vi "classify error.vi"(8 "error to classify":errorcluster, 11 "UI Reference runtime in":refnum<class "UI Reference runtime.lvclass">) -> (0 "classified error":errorcluster, 2 "error classification":T1, 3 "UI Reference runtime out":refnum<class "UI Reference runtime.lvclass">)   [LabVIEW 2014, in "UI Reference runtime.lvclass"]
doc: "Allows a module to classify an error generated at any point during execution. This <b>error classification</b> can then be used by calling code to determine if execution can continue. In addition, this function can be used to allow a component to clear an error, convert an error to a warning, or attempt to recover from an error. Recovery may be attempted only if <b>attempt recovery?</b> is true."
uses:
  UI Reference runtime.lvclass
  <vilib>/NI/Tag Bus Module Framework/runtime/error classification.ctl
  <vilib>/NI/Tag Bus Module Framework/runtime/TBM module execution interface.lvclass
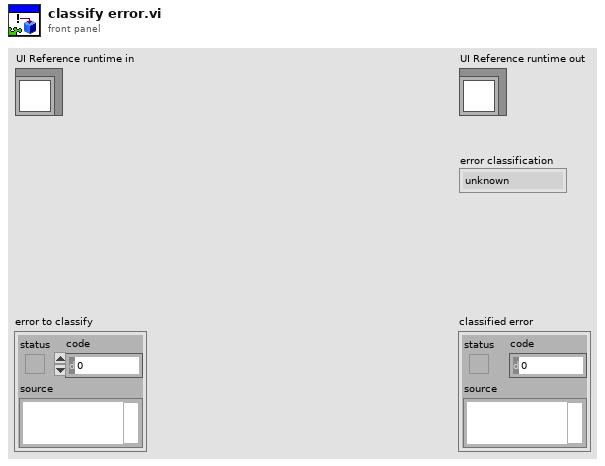
[diagram p1: front panel]
types:
  T1 = typedef "TBM module execution interface.lvclass/error classification.ctl" = enum16{"unknown", "none", "trivial", "recoverable", "critical"}
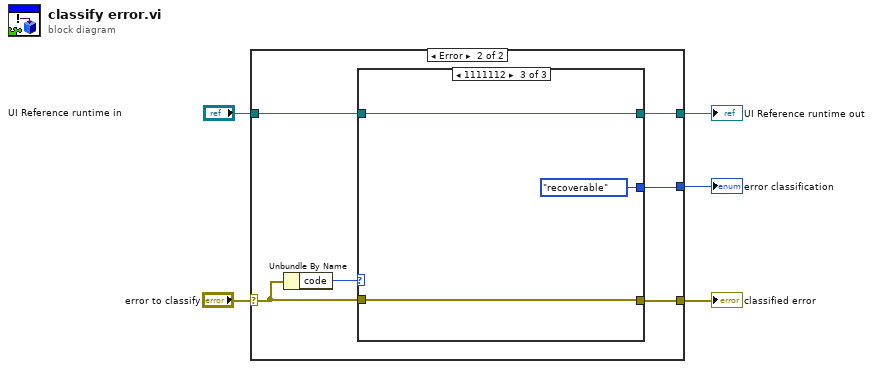
[diagram p0: block diagram]
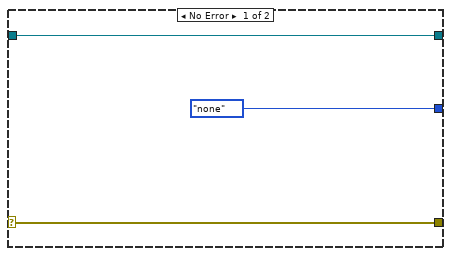
[diagram p2: hidden frame]
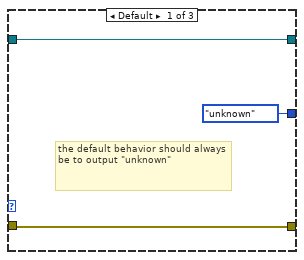
[diagram p3: hidden frame]
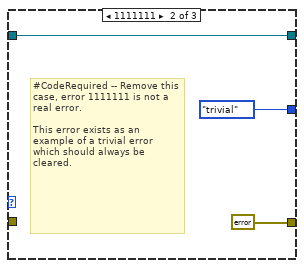
[diagram p4: hidden frame]
diagram:
  n1 = case shown="Error" "error to classify" {
    selector: "error to classify" -> [w7 w13]
    tunnel: [w8 w9] -> w4
    tunnel: "UI Reference runtime in" -> [w8 w10]
    tunnel: [w7 w12] -> w2
    tunnel: [error_classification."none" ("error classification") w11] -> w1
    frame No Error {
    }
    frame Error {
      n2 = Unbundle By Name(w13) -> ("code"=w14:i32)
      n3 = case shown="1111112" w14 {
        tunnel: w13 -> [w15 _ w23]
        tunnel: [w15 errorcluster {"status"=FALSE, "code"=0, "source"=""} ("error constant") w23] -> w12
        tunnel: [error_classification."unknown" ("error classification") error_classification."trivial" ("error classification") error_classification."recoverable" ("error classification")] -> w11
        tunnel: w10 -> [w16 w18 w21]
        tunnel: [w16 w18 w21] -> w9
        frame Default {
          # "the default behavior should always be to output \"unknown\""
        }
        frame 1111111 {
          # "#CodeRequired -- Remove this case, error 1111111 is not a real error.\n\nThis error exists as an example of a trivial error which should always be cleared."
        }
        frame 1111112 {
        }
      }
    }
  }
  "UI Reference runtime out" <- w4
  "error classification" <- w1
  "classified error" <- w2
